vi "gfitsio-get-column-size.vi"(6 "row":i32, 7 "column":string, 8 "error in (no error)":errorcluster, 11 "gfits refnum":T1) -> (0 "error out":errorcluster, 1 "variable length?":bool, 2 "nelements":i32, 3 "dup gfits refnum":T1)   [LabVIEW 2011, in "gfitsio.lvlib"]
doc: "Return number of elements in a column in an ASCII or binary table."
uses:
  gfitsio.lvlib
  gfitsio-refnum.ctl
  gfitsio.dll
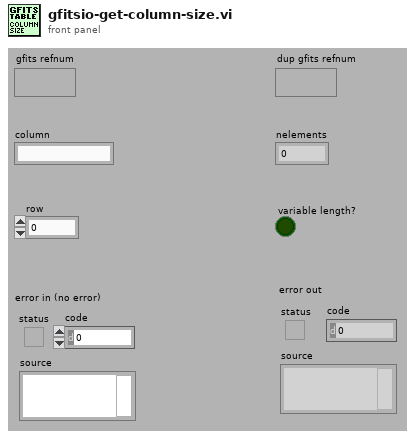
[diagram p1: front panel]
types:
  T1 = typedef "gfitsio.lvlib/gfitsio-refnum.ctl" = refnum<k1>
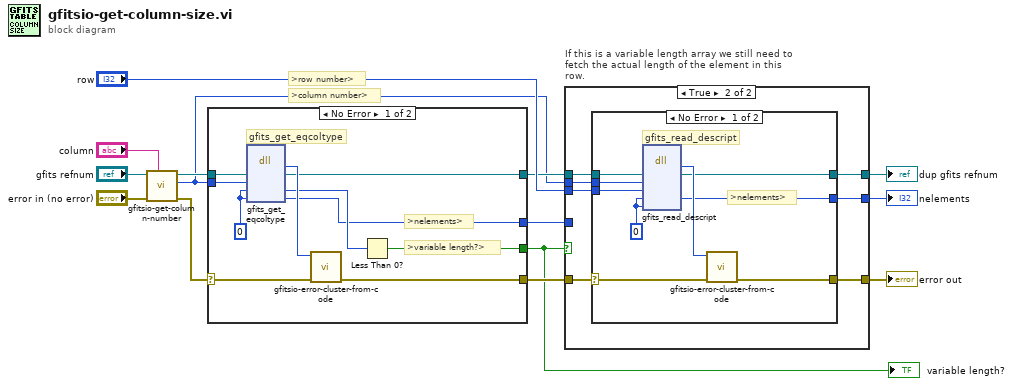
[diagram p0: block diagram]
diagram:
  # ">row number>"
  # ">column number>"
  n1 = call "gfitsio-get-column-number.vi"("column"="column", "error in (no error)"="error in (no error)", "gfits refnum"="gfits refnum") -> ("error out"=w6:errorcluster, "colnum"=w3:i32, "dup gfits refnum"=w4:T1)  [unwired: 6 in]
  n2 = case shown="No Error" w6 {
    selector: w6 -> [w23 w26]
    tunnel: [w22 w26] -> w10
    tunnel: w4 -> [w20 w25]
    tunnel: [w21 w25] -> w9
    tunnel: [w15 _] -> w1
    tunnel: w3 -> [w19 _]
    tunnel: [w18 _] -> w2
    frame No Error {
      w17 = 0
      # ">nelements>"
      # ">variable length?>"
      # "gfits_get_eqcoltype"
      n3 = dll-call lib="C:/BonOMM/BonOMM-SAOMM/SubVIs/gfitsio/gfitsio.dll" fn="gfits_get_eqcoltype"("dup gfits refnum"=w20, "colnum"=w19, "datatype"=w17, "nelements"=w17) -> (w24:i32, "dup gfits refnum"=w21:T1, "datatype"=w16:i32, "nelements"=w15:i32)  [unwired: 4 in, 2 out]
      n4 = call "gfitsio-error-cluster-from-code.vi"("error in (no error)"=w23, "error code"=w24) -> ("error out"=w22:errorcluster)  [unwired: 9 in]
      n5 = Less Than 0?(x=w16) -> (x < 0?=w18:bool)
    }
    frame Error {
    }
  }
  "variable length?" <- w2
  n6 = case "If this is a variable length array we still need to fetch the actual length of the element in this row." shown="True" w2 {
    tunnel: [w27 w36] -> w14
    tunnel: [w28 w35] -> w13
    tunnel: [w29 w34] -> w12
    tunnel: "row" -> [_ w33]
    tunnel: w10 -> [w27 w32]
    tunnel: w9 -> [w28 w31]
    tunnel: w3 -> [_ w30]
    tunnel: w1 -> [w29 _]
    frame False {
      # ">nelements>"
    }
    frame True {
      n7 = case shown="No Error" w32 {
        selector: w32 -> [w44 w47]
        tunnel: [w43 w47] -> w36
        tunnel: w31 -> [w41 w46]
        tunnel: [w42 w46] -> w35
        tunnel: [w37 _] -> w34
        tunnel: w30 -> [w40 _]
        tunnel: w33 -> [w38 _]
        frame No Error {
          w39 = 0
          # ">nelements>"
          # "gfits_read_descript"
          n8 = dll-call lib="C:/BonOMM/BonOMM-SAOMM/SubVIs/gfitsio/gfitsio.dll" fn="gfits_read_descript"("dup gfits refnum"=w41, "colnum"=w40, "row"=w38, "nelements"=w39, "offset"=w39) -> (w45:i32, "dup gfits refnum"=w42:T1, "nelements"=w37:i32)  [unwired: 6 in, 2 out]
          n9 = call "gfitsio-error-cluster-from-code.vi"("error in (no error)"=w44, "error code"=w45) -> ("error out"=w43:errorcluster)  [unwired: 9 in]
        }
        frame Error {
        }
      }
    }
  }
  "error out" <- w14
  "dup gfits refnum" <- w13
  "nelements" <- w12
